vi "Teleop.vi"(10 "Match Info":T1={"Autonomous Elapsed Seconds"=0.0, "TeleOp Elapsed Seconds"=57.34, "Disabled Elapsed Seconds"=2.708, "Visited Autonomous"=FALSE, "Visited TeleOp"=TRUE, "Visited Disabled"=TRUE, "Autonomous Settings"={"Autonomous Style"=enum."Independent", "VI Refnum"=refnum}}, 11 "Call Context":T2=enum."Execute") -> ()   [LabVIEW 2015]
doc: "This VI is called for each TeleOp packet received from the DS where the robot is not disabled. It is often used to read from the joysticks and update I/O or to update setpoints for timed control loops. It should complete and return within 20 milliseconds or it may miss DS packets."
uses:
  <vilib>/Rock Robotics/WPI/DriverStation/WPI_DriverStationDerivedRobotMode.ctl
  <vilib>/Rock Robotics/WPI/DriverStation/WPI_DriverStationMatch Info.ctl
  <vilib>/Rock Robotics/WPI/Utilities/WPI_GetSetVariantRefNum.vi
  <vilib>/Rock Robotics/Network Tables/NT Write Boolean Array.vi
  <vilib>/Rock Robotics/Network Tables/NT Write Numeric Array.vi
  <vilib>/Rock Robotics/Network Tables/NT Read Boolean.vi
  <vilib>/Rock Robotics/Network Tables/NT Read Number.vi
panel:
  in  "Intake Scale":dbl(slide)=0.2786596119929453 caption="ARM SCALE" scale=0.0..1.0
  in  "Low Shoot Scale":dbl(slide)=0.7266313932980599 caption="INTAKE SCALE" scale=0.0..1.0
  in  "DRIVE SCALE":dbl(slide)=0.4603174603174603 caption="DRIVE TRAIN SCALE" scale=0.0..1.0
  in  "ARM SCALE":dbl(slide)=0.30335097001763667 scale=0.0..1.0
  out "Sample Slider 0":dbl(slide) scale=0.0..5.0
  out "Sample Boolean 1":bool
  out "Sample Boolean 0":bool
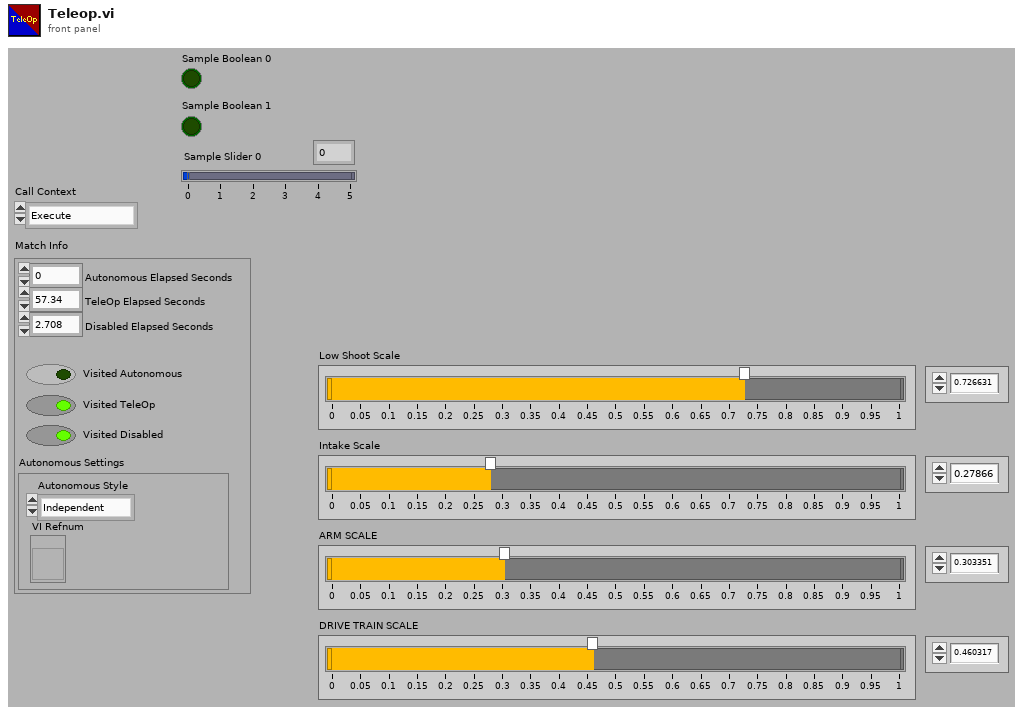
[diagram p1: front panel]
types:
  T1 = typedef "WPI_DriverStationMatch Info.ctl" = cluster{"Autonomous Elapsed Seconds":dbl, "TeleOp Elapsed Seconds":dbl, "Disabled Elapsed Seconds":dbl, "Visited Autonomous":bool, "Visited TeleOp":bool, "Visited Disabled":bool, "Autonomous Settings":cluster{"Autonomous Style":enum16{"Iterative", "Independent"}, "VI Refnum":refnum<vi>}}
  T2 = typedef "WPI_DriverStationDerivedRobotMode.ctl" = enum16{"Init", "Execute", "Stop"}
  T3 = typedef "WPI_RobotDriveDevRef.ctl" = cluster{"DevStatus":errorcluster, "Motors[]":T4[], "Square Inputs":bool, "Max Output":dbl}
  T4 = typedef "WPI_MotorControlDeviceRef.ctl" = cluster{"DeviceStatus":errorcluster, "Type":T5, "PWM":cluster{"PWM Channel":T6, "DeadBand":T7}, "CAN":cluster{"Device Number":u8, "Control Mode":T8, "Semaphore":T9, "Max Vout":dbl, "TalonSRX Control Mode":T10}, "Invert":bool}
  T5 = typedef "WPI_MotorControlType.ctl" = enum16{"PWM", "CAN", "CANTalonSRX"}
  T6 = typedef "FPGA_DIOPWMChannel.ctl" = enum8{"PWM 0", "PWM 1", "PWM 2", "PWM 3", "PWM 4", "PWM 5", "PWM 6", "PWM 7", "PWM 8", "PWM 9", "PWM MXP 0", "PWM MXP 1", "PWM MXP 2", "PWM MXP 3", "PWM MXP 4", "PWM MXP 5", "PWM MXP 6", "PWM MXP 7", "PWM MXP 8", "PWM MXP 9", "Invalid"}
  T7 = typedef "WPI_PWMDeadband.ctl" = cluster{"Name":string, "maxPositivePwm":i32, "minPositivePwm":i32, "centerPwm":i32, "maxNegativePwm":i32, "minNegativePwm":i32, "angularRange":u16}
  T8 = typedef "WPI_CANJaguar_ControlMode.ctl" = enum8{"Percent VBus", "Current", "Speed", "Position", "Voltage"}
  T9 = typedef "Semaphore RefNum" = refnum<k1>
  T10 = typedef "WPI_CANTalonSRX_APIControlMode.ctl" = enum8{"Percent VBus", "Speed", "Position", "Slave", "Unchanged / Invalid", "Voltage Compensation", "Current", "Motion Profile"}
  T11 = typedef "WPI_JoystickDevRef.ctl" = cluster{"Device":T12}
  T12 = typedef "WPI_JoystickDeviceEnum.ctl" = enum16{"USB 0", "USB 1", "USB 2", "USB 3", "USB 4", "USB 5"}
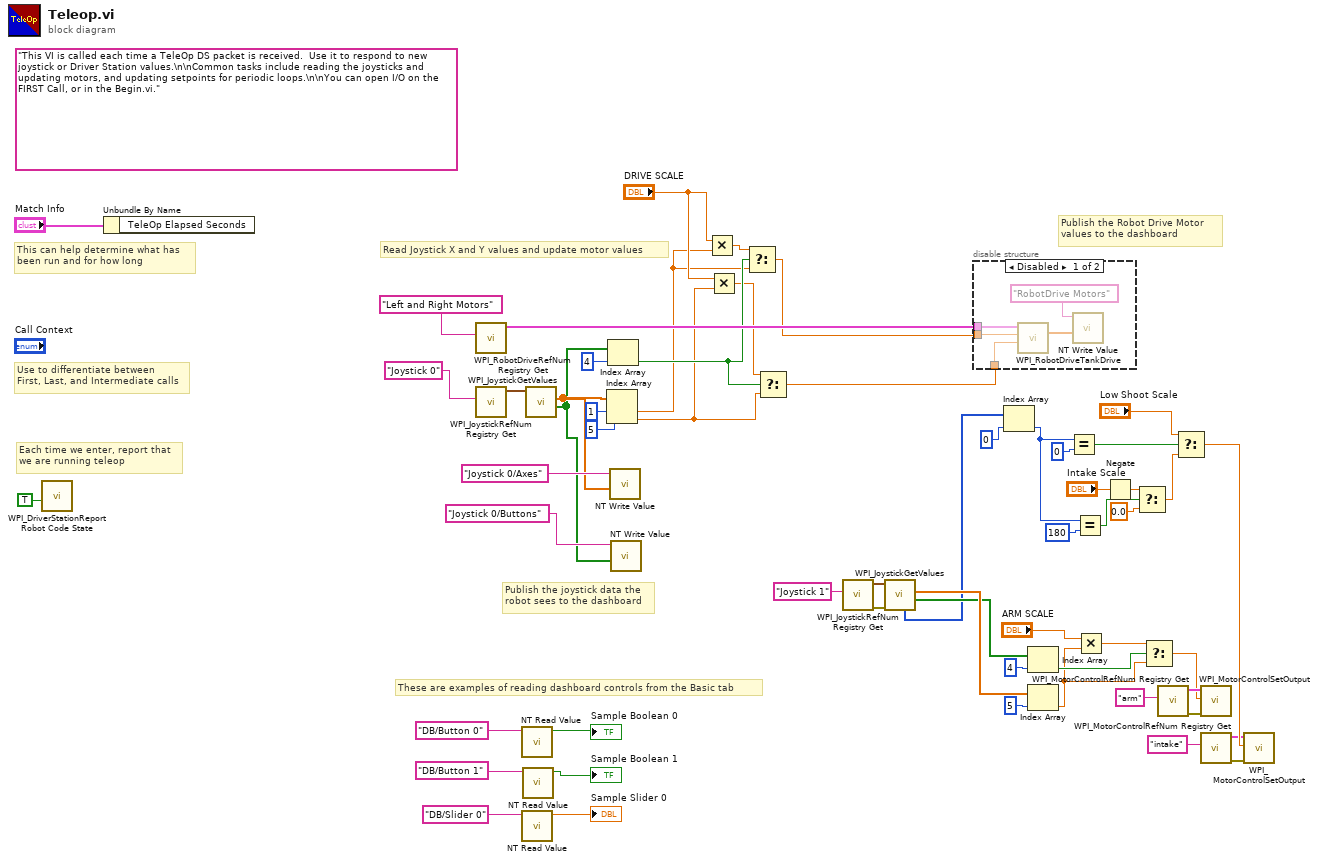
[diagram p0: block diagram]
diagram:
  (unwired) "This VI is called each time a TeleOp DS packet is received.  Use it to respond to new joystick or Driver Station values.\n\nCommon tasks include reading the joysticks and updating motors, and updating setpoints for periodic loops.\n\nYou can open I/O on the FIRST Call, or in the Begin.vi."
  # "These are examples of reading dashboard controls from the Basic tab"
  # "Publish the Robot Drive Motor\nvalues to the dashboard"
  # "Publish the joystick data the\nrobot sees to the dashboard"
  # "Each time we enter, report that\nwe are running teleop"
  # "Use to differentiate between\nFirst, Last, and Intermediate calls"
  # "This can help determine what has\nbeen run and for how long"
  # "Read Joystick X and Y values and update motor values"
  n1 = call <vilib>:"WPI_DriverStationReport Robot Code State.vi"("TeleOp"=TRUE ("Autonomous")) -> ()  [unwired: 10 in, 1 out]
  n2 = Unbundle By Name("Match Info") -> ()  [unwired: 1 out]
  n3 = call <vilib>:"WPI_RobotDriveRefNum Registry Get.vi"("refnum name"="Left and Right Motors") -> ("RobotDriveDevRef"=w56:T3)  [unwired: 1 in, 9 out]
  n4 = call <vilib>:"WPI_JoystickRefNum Registry Get.vi"("refnum name"="Joystick 0") -> ("JoystickDevRef"=w54:T11)  [unwired: 1 in, 9 out]
  n5 = call-poly <vilib>:"NT Read Value.vi"("Name"="DB/Button 0" ("refnum name")) -> ("Boolean"=→"Sample Boolean 0":bool)  [unwired: 9 in, 1 out]
  n6 = call-poly <vilib>:"NT Read Value.vi"("Name"="DB/Slider 0" ("refnum name")) -> ("Numeric"=→"Sample Slider 0":dbl)  [unwired: 9 in, 1 out]
  n7 = call-poly <vilib>:"NT Read Value.vi"("Name"="DB/Button 1" ("refnum name")) -> ("Boolean"=→"Sample Boolean 1":bool)  [unwired: 9 in, 1 out]
  n8 = call <vilib>:"WPI_JoystickGetValues.vi"("JoystickDevRef"=w54) -> ("Buttons"=w31:bool[], "Axes"=w50:dbl[])  [unwired: 6 in, 3 out]
  n9 = Index Array(array=w50, index #1=1 ("index"), index #2=5 ("index")) -> (element #1=w20:dbl, element #2=w22:dbl)
  n10 = Index Array(array=w31, index=4) -> (element=w24:bool)
  n11 = call-poly <vilib>:"NT Write Value.vi"("Numeric Array"=w50, "Name"="Joystick 0/Axes") -> ()  [unwired: 9 in, 1 out]
  n12 = call-poly <vilib>:"NT Write Value.vi"("Boolean Array"=w31, "Name"="Joystick 0/Buttons") -> ()  [unwired: 9 in, 1 out]
  n13 = Multiply(x="DRIVE SCALE", y=w20) -> (x*y=w26:dbl)
  n14 = Multiply(x="DRIVE SCALE", y=w22) -> (x*y=w23:dbl)
  n15 = Select(t=w26, s=w24, f=w20) -> (s? t:f=w27:dbl)
  n16 = Select(t=w23, s=w24, f=w22) -> (s? t:f=w21:dbl)
  n17 = call <vilib>:"WPI_JoystickRefNum Registry Get.vi"("refnum name"="Joystick 1") -> ("error out"=w36:errorcluster, "JoystickDevRef"=w37:T11)  [unwired: 1 in, 8 out]
  n18 = call <vilib>:"WPI_JoystickGetValues.vi"("error in (no error)"=w36, "JoystickDevRef"=w37) -> ("Buttons"=w18:bool[], "Axes"=w19:dbl[], "POVs"=w17:i16[])  [unwired: 5 in, 2 out]
  n19 = disable-structure shown="Disabled" {
    disable-tunnel: w56 -> [w63 _]
    disable-tunnel: w27 -> [w60 _]
    disable-tunnel: w21 -> [w59 _]
    frame Disabled {
      n20 = call <vilib>:"WPI_RobotDriveTankDrive.vi"("Right axis value"=w59, "Left axis value"=w60, "RobotDriveDevRef"=w63) -> ("Motor Values"=w62:dbl[])  [unwired: 6 in, 2 out]
      n21 = call-poly <vilib>:"NT Write Value.vi"("Numeric Array"=w62, "Name"="RobotDrive Motors") -> ()  [unwired: 9 in, 1 out]
    }
    frame Enabled {
    }
  }
  n22 = Index Array(array=w17, index=0) -> (element=w7:i16)
  n23 = Index Array(array=w18, index=4) -> (element=w33:bool)
  n24 = Index Array(array=w19, index=5) -> (element=w28:dbl)
  n25 = Equal?(x=w7, y=i16 0) -> (x = y?=w9:bool)
  n26 = Equal?(x=w7, y=i16 180) -> (x = y?=w5:bool)
  n27 = Multiply(x="ARM SCALE", y=w28) -> (x*y=w29:dbl)
  n28 = Negate(x="Intake Scale") -> (-x=w3:dbl)
  n29 = Select(t=w3, s=w5, f=0.0) -> (s? t:f=w8:dbl)
  n30 = Select(t=w29, s=w33, f=w28) -> (s? t:f=w1:dbl)
  n31 = call <vilib>:"WPI_MotorControlRefNum Registry Get.vi"("refnum name"="arm") -> ("error out"=w39:errorcluster, "MotorControlDevRef"=w40:T4)  [unwired: 9 in]
  n32 = Select(t="Low Shoot Scale", s=w9, f=w8) -> (s? t:f=w14:dbl)
  n33 = call <vilib>:"WPI_MotorControlSetOutput.vi"("error in (no error)"=w39, "Output"=w1, "MotorControlDevRef"=w40) -> ()  [unwired: 6 in, 3 out]
  n34 = call <vilib>:"WPI_MotorControlRefNum Registry Get.vi"("refnum name"="intake") -> ("error out"=w13:errorcluster, "MotorControlDevRef"=w12:T4)  [unwired: 9 in]
  n35 = call <vilib>:"WPI_MotorControlSetOutput.vi"("error in (no error)"=w13, "Output"=w14, "MotorControlDevRef"=w12) -> ()  [unwired: 6 in, 3 out]
